vi "PID Normalize Step Stimulus.vi"(7 "with initial part?":bool, 9 "Length":i32=10, 11 "Stimulus signal":dbl[](array[numeric])) -> (0 "error code":i32, 1 "Index for start step":i32, 2 "Offset":dbl, 3 "Step height":dbl)   [LabVIEW 2017, in "NI_PID_autopid.lvlib"]
uses:
  <vilib>/addons/control/pid/NI_PID_autopid.lvlib
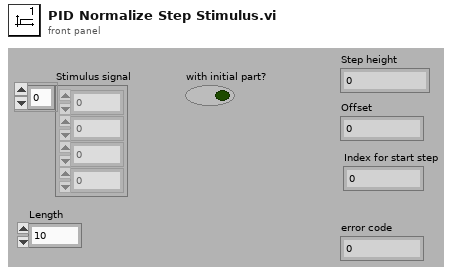
[diagram p1: front panel]
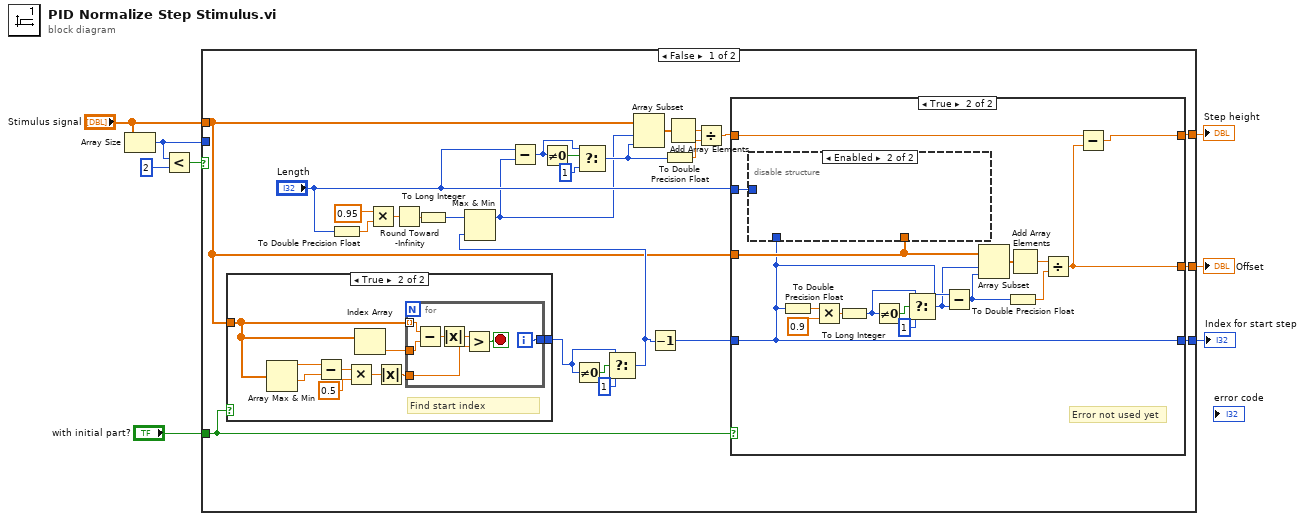
[diagram p0: block diagram]
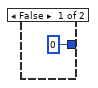
[diagram p2: hidden frame]
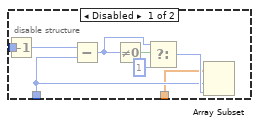
[diagram p4: hidden frame]
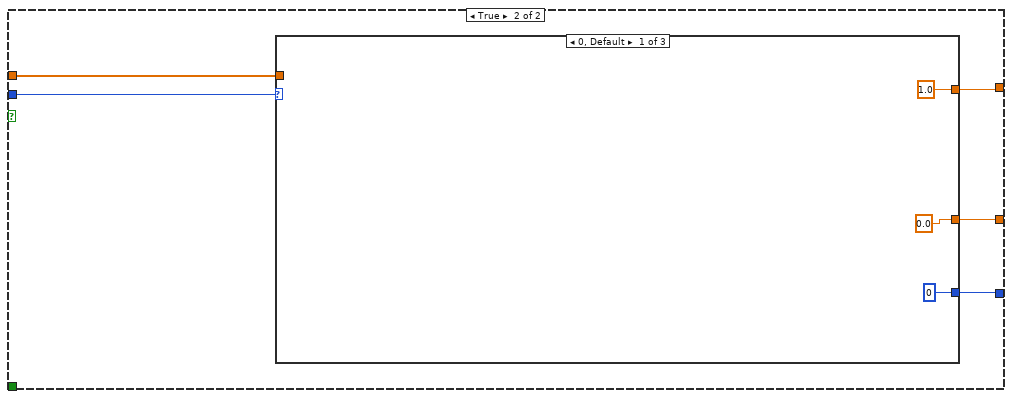
[diagram p5: hidden frame]
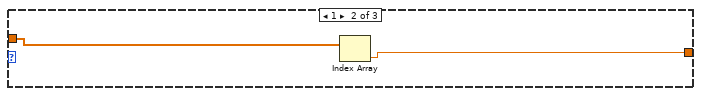
[diagram p6: hidden frame]
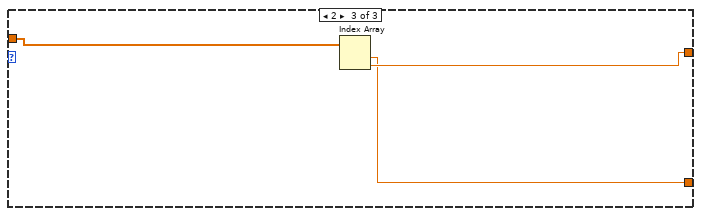
[diagram p7: hidden frame]
diagram:
  n1 = Array Size(array="Stimulus signal") -> (size(s)=w1:i32)
  n2 = Less?(x=w1, y=2) -> (x < y?=w3:bool)
  n3 = case shown="False" w3 {
    tunnel: [w33 w80] -> w8
    tunnel: [w31 w78] -> w7
    tunnel: "with initial part?" -> [w18 _]
    tunnel: [w17 w79] -> w5
    tunnel: "Stimulus signal" -> [w9 w77]
    tunnel: w1 -> [_ w81]
    frame False {
      n4 = case shown="True" w18 {
        tunnel: w9 -> [_ w36]
        tunnel: [0 w35] -> w11
        frame False {
        }
        frame True {
          # "Find start index"
          n5 = Array Max & Min(array=w36) -> (max value=w42:dbl, min value=w40:dbl)  [unwired: 2 out]
          n6 = Subtract(x=w42, y=w40) -> (x-y=w43:dbl)
          n7 = Multiply(x=w43, y=0.5) -> (x*y=w38:dbl)
          n8 = Index Array(array=w36) -> (element=w41:dbl)  [unwired: 1 in]
          n9 = Absolute Value(x=w38) -> (abs(x)=w39:dbl)
          n10 = for {
            tunnel: w36 -> [w50] mode=indexing
            tunnel: [w47] -> w35
            tunnel: w41 -> [w46]
            tunnel: w39 -> [w45]
            i -> [w47]
            stop <- w44 stop-if-true
            n11 = Subtract(x=w50, y=w46) -> (x-y=w49:dbl)
            n12 = Absolute Value(x=w49) -> (abs(x)=w48:dbl)
            n13 = Greater?(x=w48, y=w45) -> (0:w44:bool)
          }
        }
      }
      n14 = To Double Precision Float(number="Length") -> (double precision float=w25:dbl)
      n15 = Multiply(x=0.95 ("y"), y=w25) -> (x*y=w23:dbl)
      n16 = Round Toward -Infinity(1:w23) -> (0:w26:dbl)
      n17 = To Long Integer(number=w26) -> (32bit integer=w16:i32)
      n18 = Not Equal To 0?(x=w11) -> (x != 0?=w12:bool)
      n19 = Select(t=w11, s=w12, f=1) -> (s? t:f=w10:i32)
      n20 = Max & Min(x=w16, y=w10) -> (max(x,y)=w15:i32)  [unwired: 1 out]
      n21 = Subtract(x="Length", y=w15) -> (x-y=w21:i32)
      n22 = Not Equal To 0?(x=w21) -> (x != 0?=w22:bool)
      n23 = Select(t=w21, s=w22, f=1) -> (s? t:f=w19:i32)
      n24 = Array Subset(array=w9, index=w15, length=w19) -> (w27:dbl[])
      n25 = Decrement(x=w10) -> (x-1=w14:i32)
      n26 = To Double Precision Float(number=w19) -> (double precision float=w24:dbl)
      n27 = Add Array Elements(numeric array=w27) -> (sum=w30:dbl)
      n28 = Divide(x=w30, y=w24) -> (x/y=w29:dbl)
      n29 = case shown="True" w18 {
        tunnel: [w51 w55] -> w33
        tunnel: w9 -> [_ w57]
        tunnel: "Length" -> [_ w68]
        tunnel: [_ w54] -> w31
        tunnel: w29 -> [w51 w66]
        tunnel: w14 -> [_ w54]
        tunnel: [_ w56] -> w17
        frame False {
        }
        frame True {
          # "Error not used yet"
          n30 = disable-structure shown="Enabled" {
            disable-tunnel: w68 -> [w76 _]
            disable-tunnel: w54 -> [w70 _]
            disable-tunnel: w57 -> [w69 _]
            frame Disabled {
              n31 = Decrement(x=w76) -> (x-1=w75:i32)
              n32 = Subtract(x=w75, y=w70) -> (x-y=w72:i32)
              n33 = Not Equal To 0?(x=w72) -> (x != 0?=w73:bool)
              n34 = Select(t=w72, s=w73, f=1) -> (s? t:f=w71:i32)
              n35 = Array Subset(array=w69, index=w70, length=w71) -> ()  [unwired: 1 out]
            }
            frame Enabled {
            }
          }
          n36 = To Double Precision Float(number=w54) -> (double precision float=w62:dbl)
          n37 = Multiply(x=w62, y=0.9) -> (x*y=w64:dbl)
          n38 = To Long Integer(number=w64) -> (32bit integer=w58:i32)
          n39 = Not Equal To 0?(x=w58) -> (x != 0?=w60:bool)
          n40 = Select(t=w58, s=w60, f=1) -> (s? t:f=w53:i32)
          n41 = Subtract(x=w54, y=w53) -> (x-y=w52:i32)
          n42 = Array Subset(array=w57, index=w53, length=w52) -> (w63:dbl[])
          n43 = To Double Precision Float(number=w52) -> (double precision float=w61:dbl)
          n44 = Add Array Elements(numeric array=w63) -> (sum=w67:dbl)
          n45 = Divide(x=w67, y=w61) -> (x/y=w56:dbl)
          n46 = Subtract(x=w66, y=w56) -> (x-y=w55:dbl)
        }
      }
    }
    frame True {
      n47 = case shown="0, Default" w81 {
        tunnel: [1.0 w85 w88] -> w80
        tunnel: [0.0 _ w87] -> w79
        tunnel: [0 _ _] -> w78
        tunnel: w77 -> [_ w86 w89]
        frame 0, Default {
        }
        frame 1 {
          n48 = Index Array(array=w86) -> (element=w85:dbl)  [unwired: 1 in]
        }
        frame 2 {
          n49 = Index Array(array=w89) -> (element #1=w87:dbl, element #2=w88:dbl)  [unwired: 2 in]
        }
      }
    }
  }
  "Step height" <- w8
  "Index for start step" <- w7
  "Offset" <- w5
